vi "begincvlib.vi"(11 "ClearVolumeJarPath":string) -> (2 "function return":u32, 3 "ClearVolumeJarPath out":string)   [LabVIEW 2012, in "cvlib.lvlib"]
doc: "extern \"C\" __declspec(dllexport) unsigned long __cdecl begincvlib(char* ClearVolumeJarPath);"
uses:
  cvlib.lvlib
  cvlib.dll
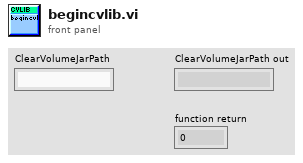
[diagram p1: front panel]
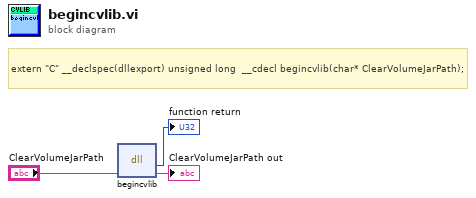
[diagram p0: block diagram]
diagram:
  # "extern \"C\" __declspec(dllexport) unsigned long \t__cdecl begincvlib(char* ClearVolumeJarPath);"
  n1 = dll-call lib="C:/Users/myerslab/workspace2/Libraries/ClearVolume/cpp/labview/lvcvlib/cvlib.*" fn="begincvlib"("ClearVolumeJarPath"="ClearVolumeJarPath") -> (→"function return":u32, "ClearVolumeJarPath"=→"ClearVolumeJarPath out":string)  [unwired: 3 in, 2 out]
